vi "sub_waypoint_save_gpx.vi"(10 "stop point index":i32[](array[numeric]), 11 "waypoint out":cluster{"x":dbl, "y":dbl}[](array[cluster])) -> (0 "error out":errorcluster, 3 "wpt":cluster{"X":dbl, "Y":dbl}[](array[cluster]))   [LabVIEW 2019]
uses:
  <vilib>/Utility/file.llb/Write Delimited Spreadsheet (DBL).vi
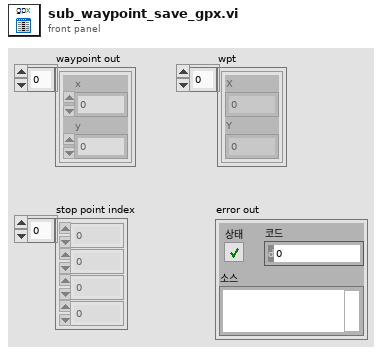
[diagram p1: front panel]
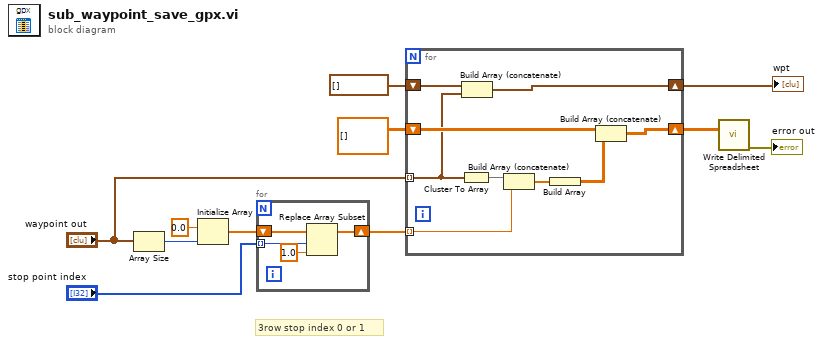
[diagram p0: block diagram]
diagram:
  # "3row stop index 0 or 1"
  n1 = Array Size(array="waypoint out") -> (size(s)=w1:i32)
  n2 = Initialize Array(0.0 ("원소"), w1) -> (w3:dbl[])
  n3 = for {
    shift-right: [w14] -> w4
    shift-left: w3 -> [w15]
    tunnel: "stop point index" -> [w13] mode=indexing
    n4 = Replace Array Subset(array=w15, new element=1.0 ("새 원소/부분배열"), index=w13) -> (w14:dbl[])
  }
  n5 = for {
    tunnel: "waypoint out" -> [w17] mode=indexing
    tunnel: w4 -> [w20] mode=indexing
    shift-right: [w21] -> w7
    shift-left: dbl[][] [] -> [w23]
    shift-right: [w16] -> w11
    shift-left: cluster{"X":dbl, "Y":dbl}[] [] -> [w18]
    n6 = Cluster To Array(cluster=w17) -> (array=w19:dbl[])
    n7 = Build Array (concatenate)(w18, w17) -> (w16:cluster{"x":dbl, "y":dbl}[])
    n8 = Build Array (concatenate)(w19, w20) -> (w24:dbl[])
    n9 = Build Array(w24) -> (w22:dbl[][])
    n10 = Build Array (concatenate)(w23, w22) -> (w21:dbl[][])
  }
  "wpt" <- w11
  n11 = call-poly <vilib>:"Write Delimited Spreadsheet.vi"("2D data"=w7) -> ("error out"=→"error out":errorcluster)  [unwired: 13 in, 1 out]
